vi "NewTrace.vi"(0 "VISA IN":refnum<visa-resource-name>, 1 "Measurement":string(combo)="S21", 2 "FileName":string="Test", 3 "Window":i32=1, 4 "Trace":i32=2, 5 "error in (no error)":errorcluster, 7 "Channel":i32=1) -> (14 "VISA Out":refnum<visa-resource-name>, 19 "error out":errorcluster)   [LabVIEW 2018, in "PNA-X.lvlib"]
uses:
  PNA-X.lvlib
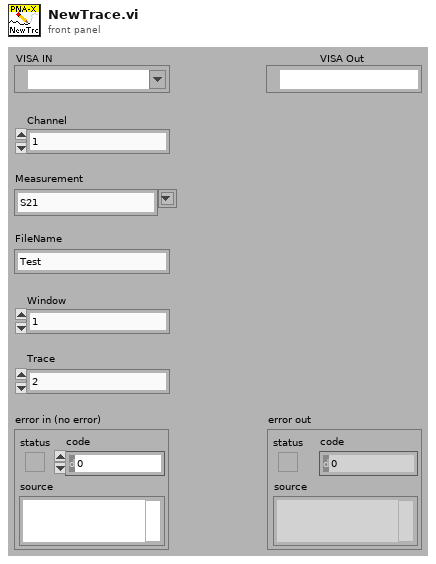
[diagram p1: front panel]
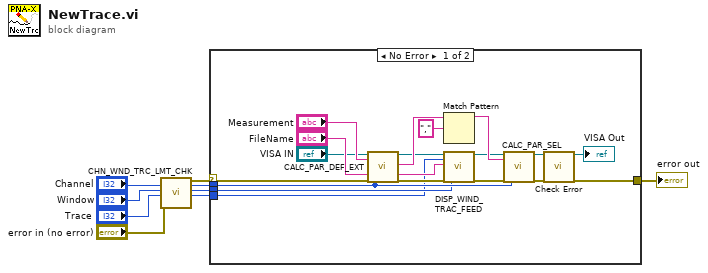
[diagram p0: block diagram]
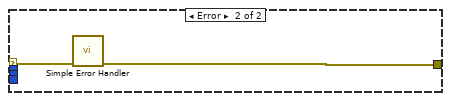
[diagram p2: hidden frame]
diagram:
  n1 = call "CHN_WND_TRC_LMT_CHK.vi"("Channel"="Channel", "Window"="Window", "Trace"="Trace", "error in"="error in (no error)") -> ("error out"=w8:errorcluster, "Channel"=w3:i32, "Window"=w2:i32, "Trace"=w1:i32)  [unwired: 11 in, 1 out]
  n2 = case shown="No Error" w8 {
    selector: w8 -> [w18 w30]
    tunnel: [w28 w29] -> w9
    tunnel: w3 -> [w12 _]
    tunnel: w2 -> [w11 _]
    tunnel: w1 -> [w10 _]
    frame No Error {
      n3 = call "CALC_PAR_DEF_EXT.vi"("VISA IN"="VISA IN", "Measurement Name"="Measurement", "FileName"="FileName", "error in"=w18, "Channel"=w12) -> ("VISA Out"=w16:refnum<visa-resource-name>, "Meas"=w21:string, "FileName"=w20:string, "error out"=w14:errorcluster)  [unwired: 11 in]
      n4 = Match Pattern(string=w21, regular expression=",") -> (before substring=w23:string)  [unwired: 1 in, 3 out]
      n5 = call "DISP_WIND_TRAC_FEED.vi"("VISA IN"=w16, "Trace"=w10, "Name"=w20, "error in"=w14, "Window"=w11) -> ("VISA Out"=w15:refnum<visa-resource-name>, "error out"=w13:errorcluster)  [unwired: 13 in]
      n6 = call "CALC_PAR_SEL.vi"("VISA IN"=w15, "Measurement"=w23, "error in"=w13, "Channel"=w12) -> ("VISA Out"=w22:refnum<visa-resource-name>, "error out"=w25:errorcluster)  [unwired: 14 in]
      n7 = call "Check Error.vi"("VISA Resource Name"=w22, "error in (no error)"=w25) -> ("dup VISA session"=→"VISA Out":refnum<visa-resource-name>, "error out"=w28:errorcluster)  [unwired: 16 in]
    }
    frame Error {
      n8 = call <vilib>:"Simple Error Handler.vi"("error in (no error)"=w30) -> ("error out"=w29:errorcluster)  [unwired: 4 in, 4 out]
    }
  }
  "error out" <- w9
